vi "ModifyUser.vi"() -> ()   [LabVIEW 2013]
doc: "This VI is the solution to Exercise 3-1 of the LabVIEW Basics II course.\n\nThis VI will accept a user name and password, and after the OK button is pressed, verify if the information is valid using the Verify Information subVI. The name and password controls are initialized to empty strings and the Key Focus attribute of the Login Name control is set to TRUE.\n\nYou will use this VI in Application Exercise.vi (Exercise 5-1) as your login screen."
uses:
  SourceCode/GlobalValue.vi
  <vilib>/Utility/config.llb/Write Key (String).vi
  <vilib>/Utility/config.llb/NI_LVConfig.lvlib
panel:
  out "error out":errorcluster caption="错误输出"
  in  "error in (no error)":errorcluster
  in  "Cancle":bool
  in  "save":bool
  in  "Password":string
  in  "用户名":string
  # "修改用户名和密码"
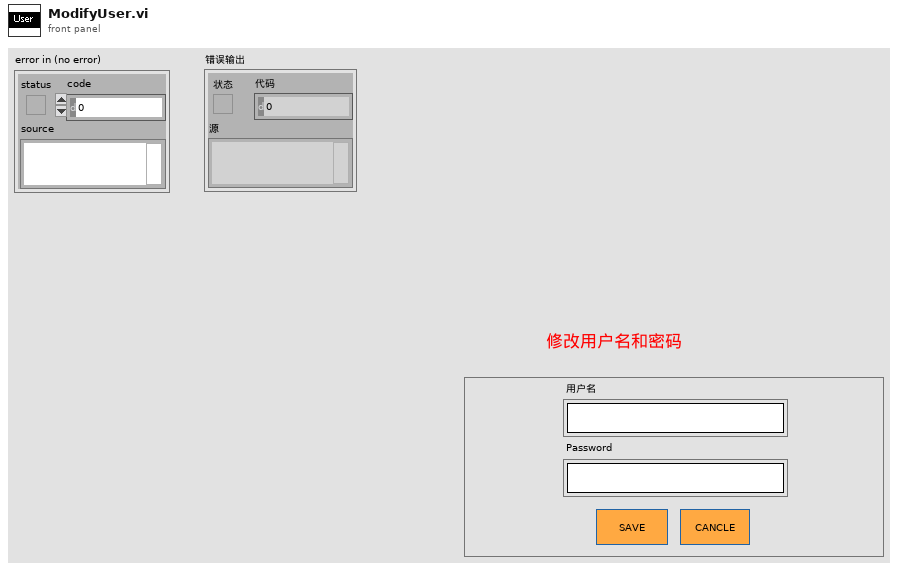
[diagram p1: front panel]
types:
  T1 = typedef "NI_LVConfig.lvlib/Config Data RefNum.ctl" = refnum<k1>
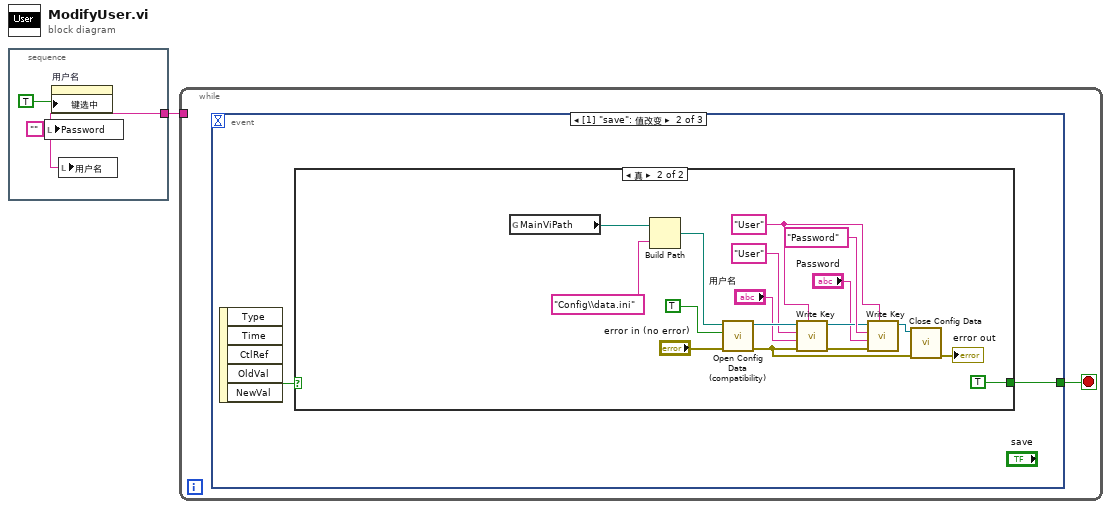
[diagram p0: block diagram]
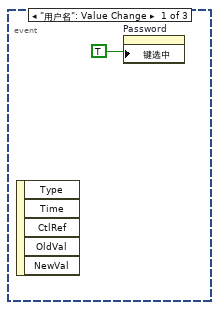
[diagram p2: hidden frame]
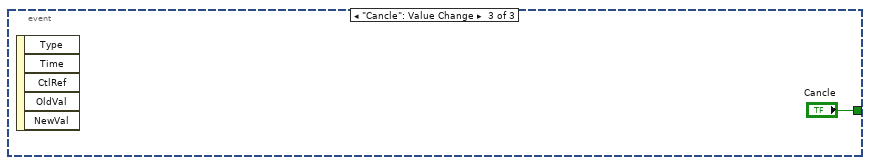
[diagram p4: hidden frame]
diagram:
  n1 = stacked-sequence {
    tunnel: [w2] -> w1
    frame #0 {
      w2 = ""
      n2 = local write "Password"(w2) -> ()
      n3 = property on="用户名" class="Str"("键选中"=TRUE ("Key Focus")) -> ()  [unwired: 2 in, 2 out]
      n4 = local write "用户名"(w2) -> ()
    }
  }
  n5 = while {
    tunnel: w1 -> [_]
    stop <- w4 stop-if-true
    n6 = event shown="[1] \"save\": 值改变" {
      selector: _ -> [_ _ _]
      dyn-events: _ -> [_ _ _]
      timeout: _ -> [_ _ _]
      tunnel: [_ w6 "Cancle"] -> w4
      event "用户名": Value Change {
        n7 = event-data() -> ()  [unwired: 6 out]
        n8 = property on="Password" class="Str"("键选中"=TRUE ("Key Focus")) -> ()  [unwired: 2 in, 2 out]
      }
      event "save": Value Change {
        n9 = event-data() -> ("NewVal"=w7:bool)  [unwired: 5 out]
        n10 = case shown="真" w7 {
          tunnel: [_ TRUE] -> w6
          frame False {
          }
          frame True {
            w20 = "User" ("ModelName")
            n11 = global read "GlobalValue.vi" "MainViPath"() -> (w8:path)
            n12 = Build Path(base path=w8, name or relative path="Config\\data.ini" ("名称或相对路径")) -> (appended path=w15:path)
            n13 = call <vilib>:"Open Config Data (compatibility).vi"("error in (no error)"="error in (no error)", "create file if necessary (T)"=TRUE, "configuration file path"=w15) -> ("error out"=w24:errorcluster, "refnum"=w22:T1)  [unwired: 6 in, 1 out]
            n14 = call-poly <vilib>:"Write Key.vi"("section"=w20, "error in (no error)"=w24, "value"="用户名", "key"="User", "refnum"=w22) -> ("error out"=w19:errorcluster, "refnum out"=w18:T1)  [unwired: 1 in, 4 out]
            n15 = call-poly <vilib>:"Write Key.vi"("section"=w20, "error in (no error)"=w19, "value"="Password", "key"="Password", "refnum"=w18) -> ("refnum out"=w23:T1)  [unwired: 1 in, 5 out]
            n16 = call <vilib>:"Close Config Data.vi"("error in (no error)"=w24, "refnum"=w23) -> ("error out"=→"error out":errorcluster)  [unwired: 1 in, 8 out]
          }
        }
      }
      event "Cancle": Value Change {
        n17 = event-data() -> ()  [unwired: 6 out]
      }
    }
  }
